vi "DependencyViewer_Configuration.vi"(8 "error in":errorcluster, 11 "ProjectPath":path) -> (0 "error out":errorcluster)   [LabVIEW 2020]
uses:
  DependencyChecker/FilterOptions.ctl
  DependencyChecker/Settings.ctl
  DependencyChecker/DependencyConfiguration.ctl
  <vilib>/Utility/sysdir.llb/System Directory Type.ctl
  DP-Common/DP-Common.lvlib
  DependencyViewer/DependencyViewer.lvlib
panel:
  in  "Max reports to save":u8 min=1
  in  "Close":bool
  in  "SaveChanges":bool
  in  "IgnoreLibrariesInCircularDependencies":bool
  in  "OnlyKeepCircularDepedencies":bool
  in  "Filter Options":T1={"Ignore user.lib"=FALSE, "Ignore vi.lib"=FALSE, "Ignore instr.lib"=FALSE, "FolderToIgnore"=[], "Ignore libraries"=FALSE, "Ignore lvcasses"=FALSE, "Ignore xnodes"=TRUE, "Ignore xcontrols"=TRUE, "Ignore Channel Classes"=TRUE}
  in  "RemoveEvenSubLibraries":bool
  in  "RemoveItemsBelongingToLibraries":bool
  in  "OpenFolder":bool
  in  "EmbedChartScript":bool
  in  "Remove Configuration":bool
  in  "Dependency configuration name":string
  in  "Add Configuration":bool
  in  "_ShowContextHelp":bool
  in  "Help":bool
  in  "Revert":bool
  in  "Update":bool
  in  "Dependency configurations":i32(listbox) caption="Will show up in the right click menu"
  in  "UseProjectFolder":bool
  in  "Folder to save reports to":path caption="Folder to save reports to (Absolute)"
  # "Dependency Viewer Configuration"
  # "Filter option for configuration"
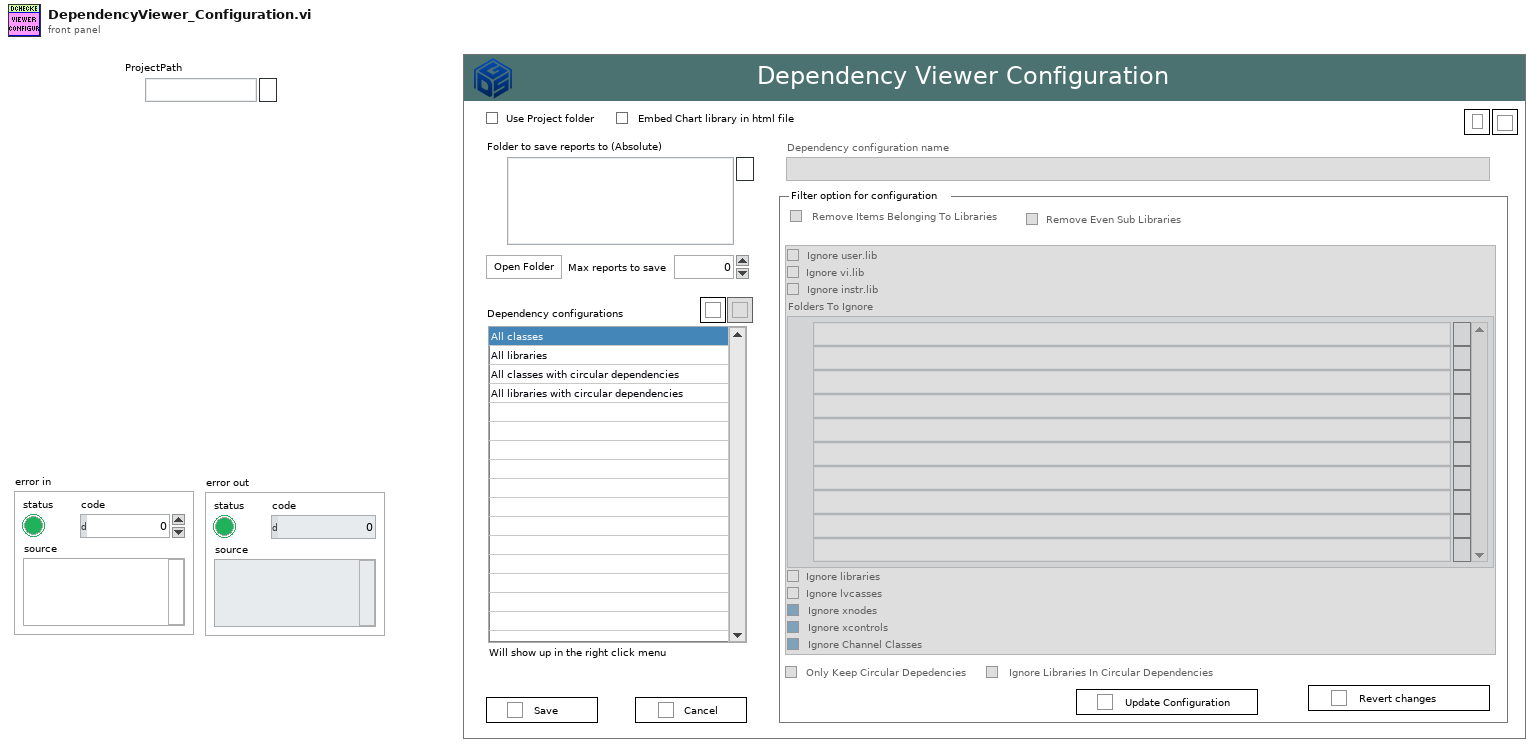
[diagram p1: front panel]
types:
  T1 = typedef "DependencyViewer.lvlib/FilterOptions.ctl" = cluster{"Ignore user.lib":bool, "Ignore vi.lib":bool, "Ignore instr.lib":bool, "FolderToIgnore":path[], "Ignore libraries":bool, "Ignore lvcasses":bool, "Ignore xnodes":bool, "Ignore xcontrols":bool, "Ignore Channel Classes":bool}
  T2 = typedef "System Directory Type.ctl" = i32
  T3 = typedef "DependencyViewer.lvlib/Settings.ctl" = cluster{"EmbedChartLibraryScript":bool, "Configurations":T4[], "UseProjectFolder":bool, "Folder to save reports to":path, "Max reports to save":u8}
  T4 = typedef "DependencyViewer.lvlib/DependencyConfiguration.ctl" = cluster{"Name":string, "RemoveItemsBelongingToLibraries":bool, "RemoveEvenSubLibraries":bool, "FilterOptions":T1, "OnlyKeepCircularDepedencies":bool, "IgnoreLibrariesInCircularDependencies":bool}
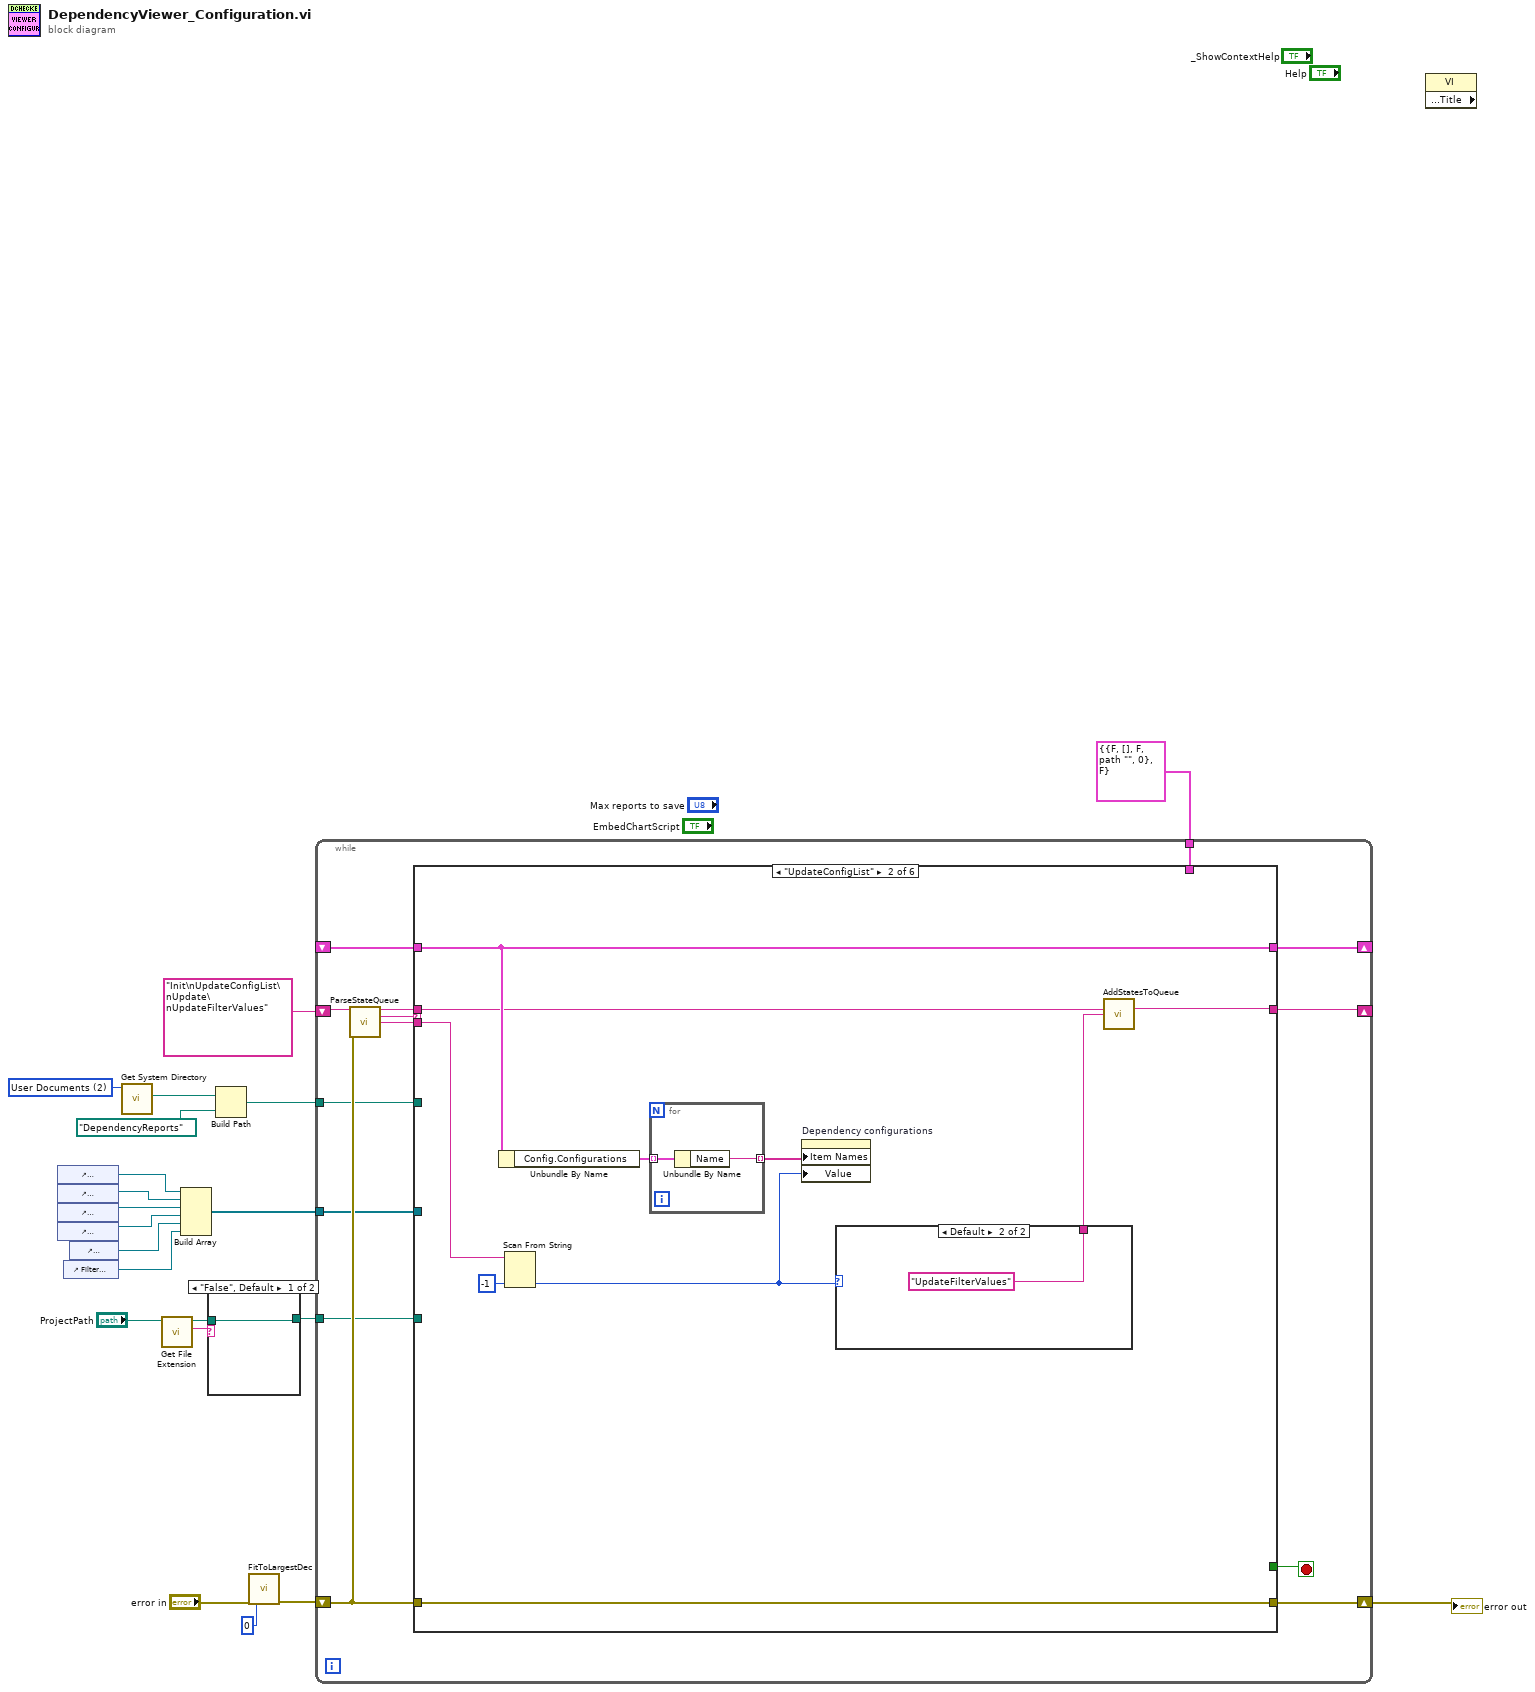
[diagram p0: block diagram]
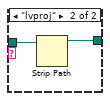
[diagram p2: hidden frame]
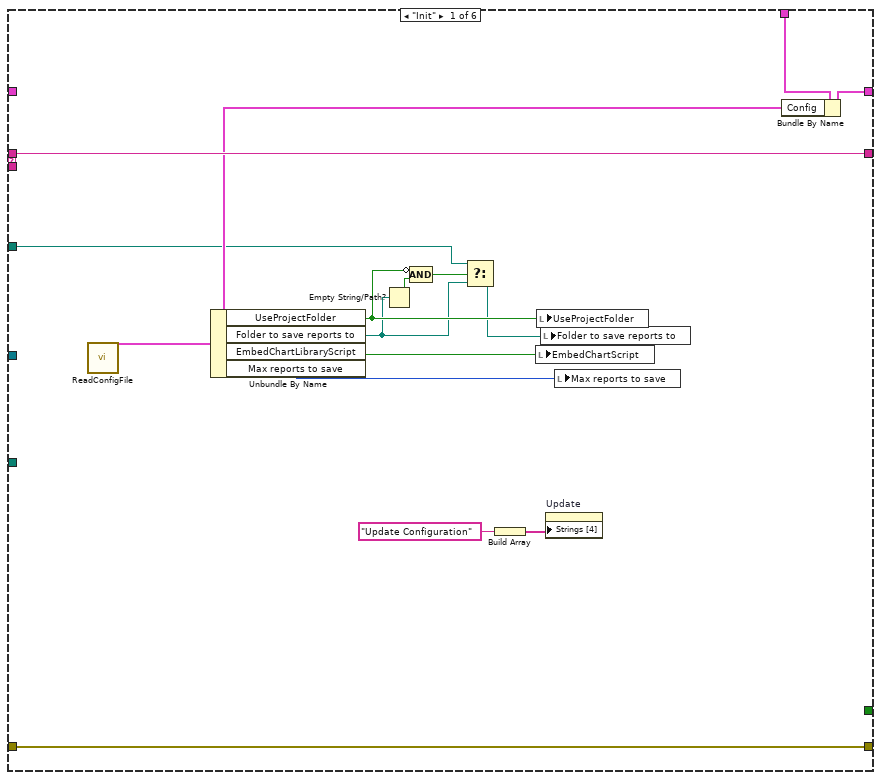
[diagram p3: hidden frame]
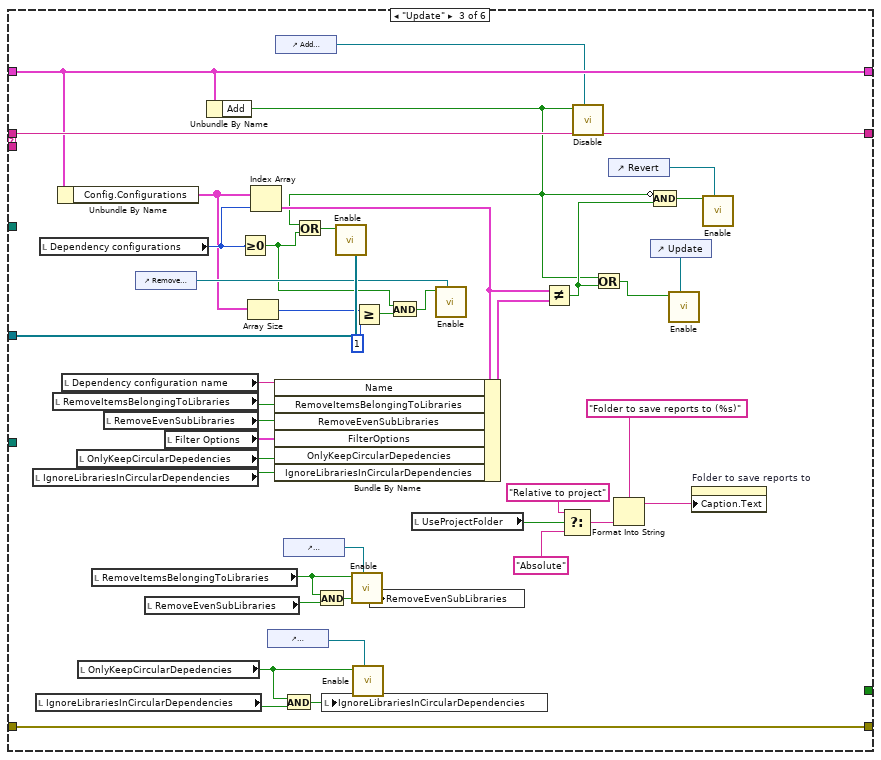
[diagram p5: hidden frame]
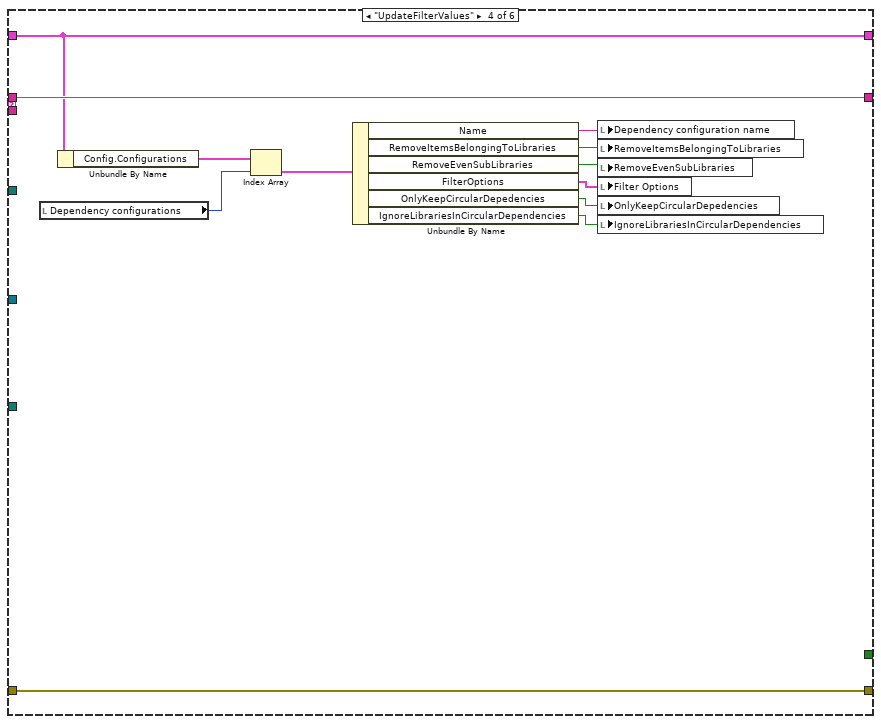
[diagram p6: hidden frame]
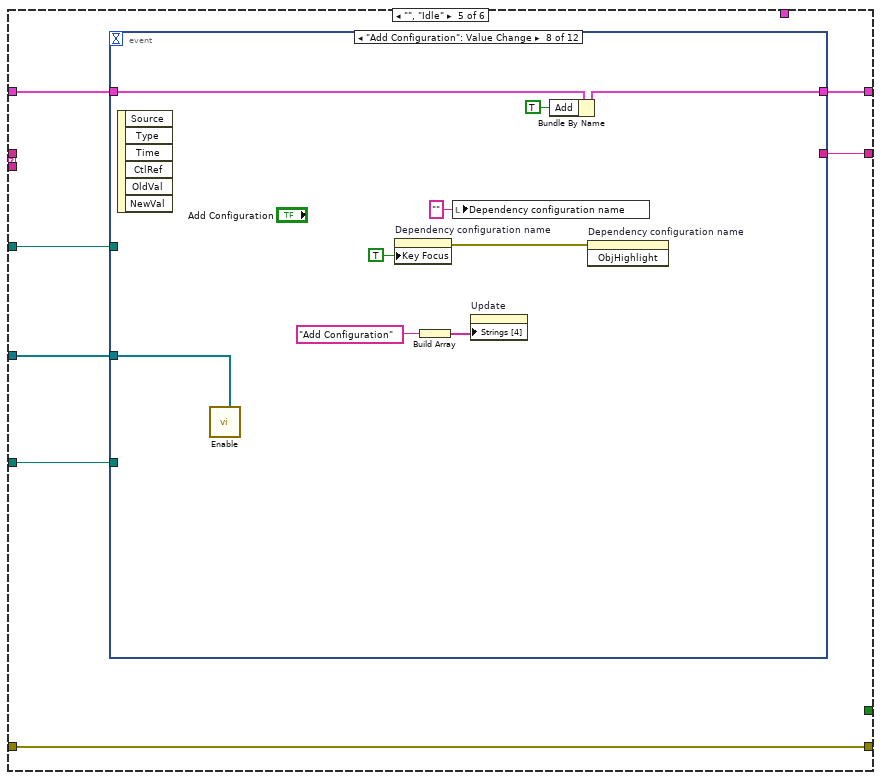
[diagram p7: hidden frame]
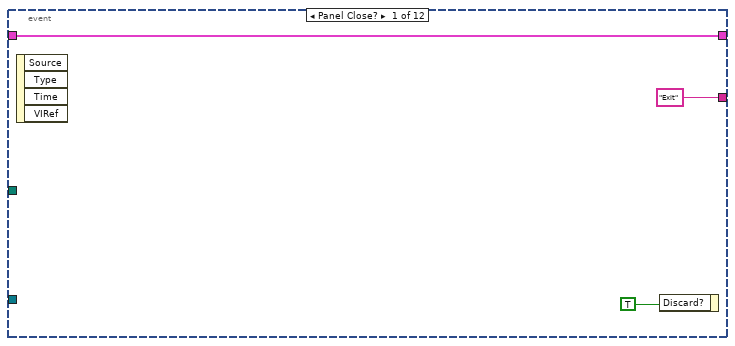
[diagram p8: hidden frame]
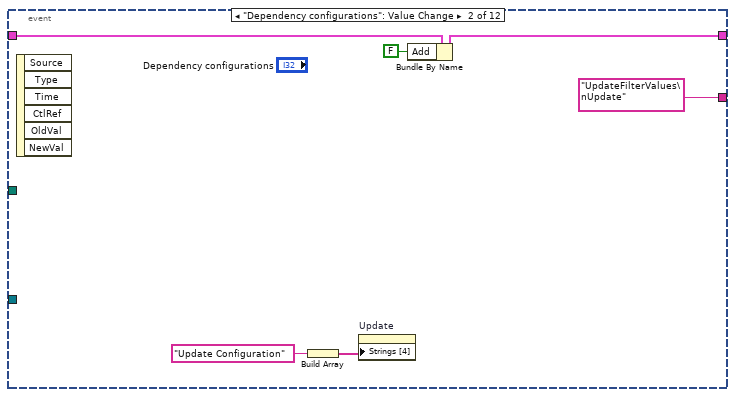
[diagram p9: hidden frame]
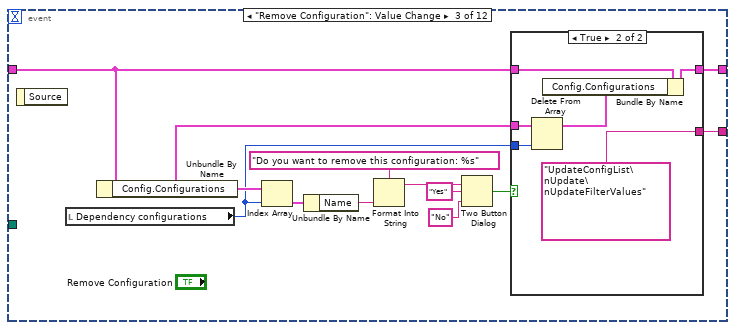
[diagram p10: hidden frame]
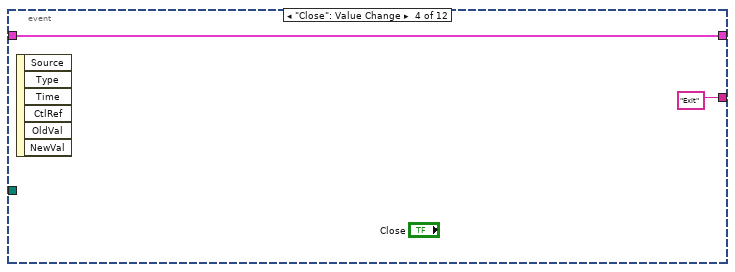
[diagram p12: hidden frame]
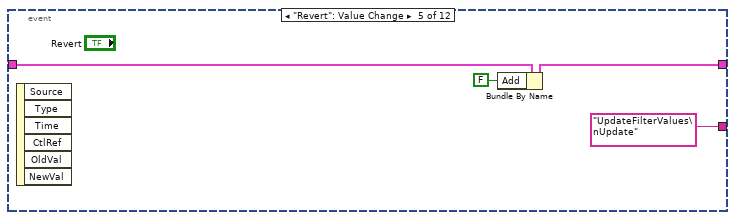
[diagram p13: hidden frame]
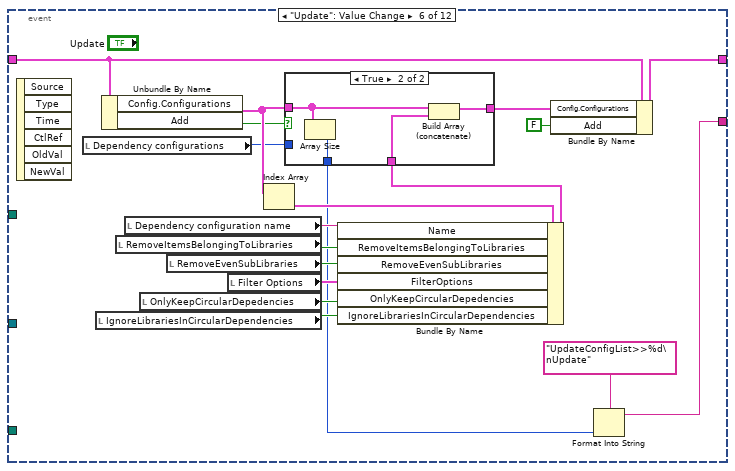
[diagram p14: hidden frame]
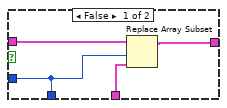
[diagram p15: hidden frame]
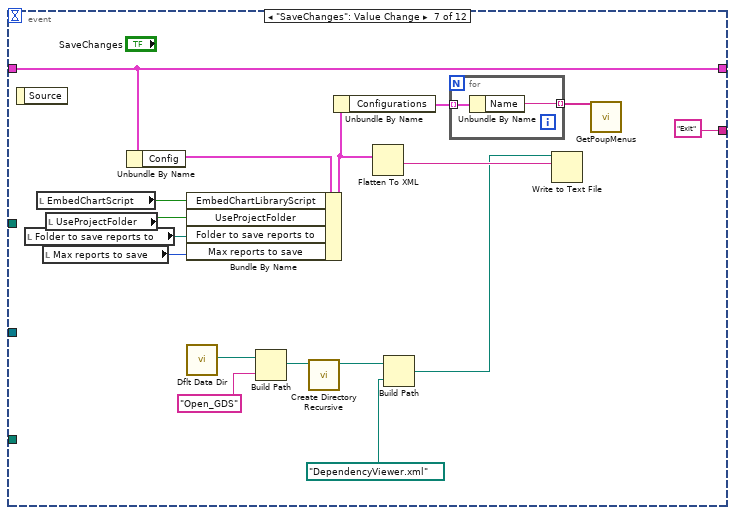
[diagram p16: hidden frame]
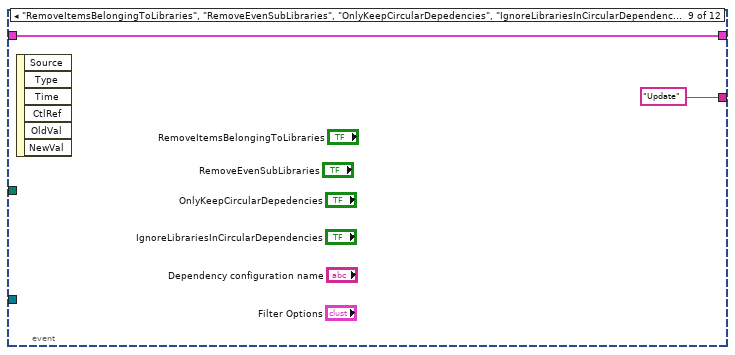
[diagram p17: hidden frame]
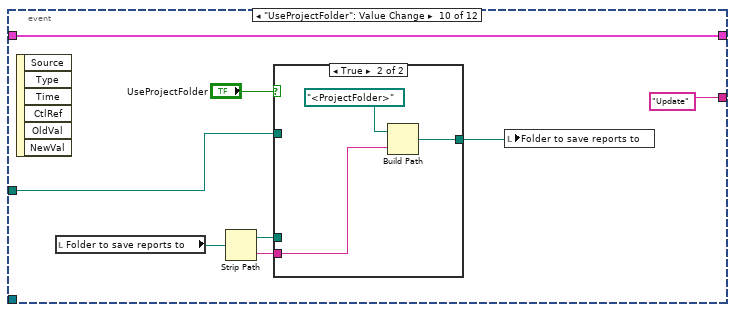
[diagram p18: hidden frame]
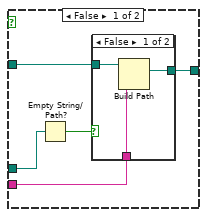
[diagram p19: hidden frame]
diagram:
  w8 = T2 2 items=["User Home"=0, "User Desktop"=1, "User Documents"=2, "User Application Data"=3, "User Preferences"=4, "User Temporary"=5, "Public Documents"=6, "Public Application Data"=7, "Public Preferences"=8, "Public Cache"=13, "System Core Libraries"=9, "System Installed Libraries"=10, "Application Files"=11, "Boot Volume Root"=12] ("system directory type")
  n1 = control-ref of="IgnoreLibrariesInCircularDependencies"() -> (w16:refnum<vi>)
  n2 = control-ref of="OnlyKeepCircularDepedencies"() -> (w15:refnum<vi>)
  n3 = control-ref of="RemoveEvenSubLibraries"() -> (w14:refnum<vi>)
  n4 = control-ref of="RemoveItemsBelongingToLibraries"() -> (w13:refnum<vi>)
  n5 = control-ref of="Filter Options"() -> (w11:refnum<vi>)
  n6 = control-ref of="Dependency configuration name"() -> (w12:refnum<vi>)
  n7 = call <vilib>:"Get System Directory.vi"("system directory type"=w8) -> ("system directory"=w7:path)  [unwired: 10 in]
  n8 = call <vilib>:"Get File Extension.vi"("file"="ProjectPath") -> ("lowercase file extension"=w3:string, "dup file"=w2:path)  [unwired: 6 in, 3 out]
  n9 = Build Array(w16, w15, w14, w13, w12, w11) -> (w10:refnum<vi>[])
  n10 = case shown="\"False\", Default" w3 {
    tunnel: w2 -> [w22 w24]
    tunnel: [w22 w23] -> w1
    frame "False", Default {
    }
    frame "lvproj" {
      n11 = Strip Path(path=w24) -> (stripped path=w23:path)  [unwired: 1 out]
    }
  }
  n12 = Build Path(base path=w7, name or relative path=path "DependencyReports") -> (appended path=w5:path)
  n13 = call "FitToLargestDec.vi"("error in (no error)"="error in", "border spacing (2 px)"=0) -> ("error out"=w17:errorcluster)  [unwired: 4 in, 1 out]
  n14 = while {
    shift-right: [w33] -> _
    shift-left: "Init\nUpdateConfigList\nUpdate\nUpdateFilterValues" -> [w38]
    shift-right: [w35] -> w19
    shift-left: w17 -> [w36]
    tunnel: cluster{"Config":T3, "Add":bool} {"Config"={"EmbedChartLibraryScript"=FALSE, "Configurations"=[], "UseProjectFolder"=FALSE, "Folder to save reports to"=path "", "Max reports to save"=0}, "Add"=FALSE} -> [w31]
    shift-right: [w30] -> _
    shift-left: _ -> [w29]
    tunnel: w10 -> [w27]
    tunnel: w5 -> [w26]
    tunnel: w1 -> [w25]
    stop <- w32 stop-if-true
    n15 = call "ParseStateQueue.vi"("State Queue"=w38, "Error In (no error)"=w36) -> ("Remaining States"=w34:string, "Current State"=w37:string, "Arguments"=w28:string)  [unwired: 9 in, 2 out]
    n16 = case shown="\"UpdateConfigList\"" w37 {
      tunnel: w36 -> [w53 w63 w99 w119 w127 w266]
      tunnel: [w53 w63 w99 w119 w127 w266] -> w35
      tunnel: [w52 w56 w100 w120 w124 w268] -> w33
      tunnel: w34 -> [w52 w57 w100 w120 _ w268]
      tunnel: [_ _ _ _ _ TRUE] -> w32
      tunnel: w31 -> [w51 _ _ _ _ _]
      tunnel: [w50 w61 w81 w118 w125 w265] -> w30
      tunnel: w29 -> [_ w61 w81 w118 w126 w265]
      tunnel: w28 -> [_ w59 _ _ _ _]
      tunnel: w27 -> [_ _ w97 _ w121 _]
      tunnel: w26 -> [w39 _ _ _ w123 _]
      tunnel: w25 -> [_ _ _ _ w122 _]
      frame "Init" {
        n17 = call "ReadConfigFile.vi"() -> ("Config"=w49:T3)  [unwired: 11 in]
        n18 = Unbundle By Name(w49) -> ("UseProjectFolder"=w44:bool, "Folder to save reports to"=w41:path, "EmbedChartLibraryScript"=w48:bool, "Max reports to save"=w45:u8)
        n19 = Empty String/Path?(string/path=w41) -> (empty?=w43:bool)
        n20 = Compound Arithmetic op=AND(invert w44, w43) -> (w42:bool)
        n21 = Select(t=w39, s=w42, f=w41) -> (s? t:f=w40:path)
        n22 = Build Array("Update Configuration") -> (w47:string[])
        n23 = local write "EmbedChartScript"(w48) -> ()
        n24 = local write "UseProjectFolder"(w44) -> ()
        n25 = local write "Folder to save reports to"(w40) -> ()
        n26 = property on="Update" class="Bool"("Strings [4]"=w47) -> ()  [unwired: 2 in, 2 out]
        n27 = local write "Max reports to save"(w45) -> ()
        n28 = Bundle By Name(cluster=w51, "Config"=w49) -> (w50:cluster{"Config":T3, "Add":bool})
      }
      frame "UpdateConfigList" {
        n29 = Unbundle By Name(w61) -> ("Config.Configurations"=w62:T4[])
        n30 = Scan From String(input string=w59, default 1=-1 ("default value 1")) -> (output 1=w55:i32)  [unwired: 3 in, 3 out]
        n31 = for {
          tunnel: w62 -> [w66] mode=indexing
          tunnel: [w65] -> w60 mode=indexing
          n32 = Unbundle By Name(w66) -> ("Name"=w65:string)
        }
        n33 = property on="Dependency configurations" class="LstBox (strict)"("Item Names"=w60, "Value"=w55) -> ()  [unwired: 2 in, 2 out]
        n34 = case shown="Default" w55 {
          tunnel: [_ "UpdateFilterValues"] -> w54
          frame -1 {
          }
          frame Default {
          }
        }
        n35 = call "AddStatesToQueue.vi"("State(s) in (\"\")"=w57, "State(s) at Back (\"\")"=w54) -> ("States Out"=w56:string)  [unwired: 13 in]
      }
      frame "Update" {
        n36 = local read "IgnoreLibrariesInCircularDependencies"() -> (w90:bool)
        n37 = local read "IgnoreLibrariesInCircularDependencies"() -> (w102:bool)
        n38 = local read "Dependency configurations"() -> (w98:i32)
        n39 = local read "RemoveItemsBelongingToLibraries"() -> (w94:bool)
        n40 = Unbundle By Name(w81) -> ("Config.Configurations"=w87:T4[])
        n41 = local read "Dependency configuration name"() -> (w95:string)
        n42 = local read "OnlyKeepCircularDepedencies"() -> (w91:bool)
        n43 = local read "OnlyKeepCircularDepedencies"() -> (w103:bool)
        n44 = local read "RemoveItemsBelongingToLibraries"() -> (w106:bool)
        n45 = local read "RemoveEvenSubLibraries"() -> (w93:bool)
        n46 = control-ref of="Remove Configuration"() -> (w96:refnum<vi>)
        n47 = local read "RemoveEvenSubLibraries"() -> (w107:bool)
        n48 = local read "Filter Options"() -> (w92:T1)
        n49 = Unbundle By Name(w81) -> ("Add"=w68:bool)
        n50 = Greater Or Equal To 0?(x=w98) -> (x >= 0?=w72:bool)
        n51 = Array Size(array=w87) -> (size(s)=w86:i32)
        n52 = Index Array(array=w87, index=w98) -> (element=w88:T4)
        n53 = control-ref of="IgnoreLibrariesInCircularDependencies"() -> (w104:refnum<vi>)
        n54 = Bundle By Name(cluster=w88, "Name"=w95, "RemoveItemsBelongingToLibraries"=w94, "RemoveEvenSubLibraries"=w93, "FilterOptions"=w92, "OnlyKeepCircularDepedencies"=w91, "IgnoreLibrariesInCircularDependencies"=w90) -> (w89:T4)
        n55 = control-ref of="Add Configuration"() -> (w67:refnum<vi>)
        n56 = control-ref of="RemoveEvenSubLibraries"() -> (w108:refnum<vi>)
        n57 = And(x=w103, y=w102) -> (x .and. y?=w101:bool)
        n58 = Or(x=w68, y=w72) -> (x .or. y?=w71:bool)
        n59 = And(x=w106, y=w107) -> (x .and. y?=w105:bool)
        n60 = local write "IgnoreLibrariesInCircularDependencies"(w101) -> ()
        n61 = call "Enable.vi"("ManyControls"=w97, "Enable(True)"=w71) -> ()  [unwired: 9 in, 1 out]
        n62 = call "Enable.vi"("ControlRefnum(IgnoreIfNotWired)"=w108, "Enable(True)"=w106) -> ()  [unwired: 9 in, 1 out]
        n63 = call "Enable.vi"("ControlRefnum(IgnoreIfNotWired)"=w104, "Enable(True)"=w103) -> ()  [unwired: 9 in, 1 out]
        n64 = Greater Or Equal?(x=w86, y=1) -> (x >= y?=w84:bool)
        n65 = local write "RemoveEvenSubLibraries"(w105) -> ()
        n66 = And(x=w72, y=w84) -> (x .and. y?=w83:bool)
        n67 = local read "UseProjectFolder"() -> (w77:bool)
        n68 = call "Enable.vi"("ControlRefnum(IgnoreIfNotWired)"=w96, "Enable(True)"=w83) -> ()  [unwired: 9 in, 1 out]
        n69 = Not Equal?(x=w88, y=w89) -> (x != y?=w70:bool)
        n70 = Select(t="Relative to project", s=w77, f="Absolute") -> (s? t:f=w76:string)
        n71 = call "Disable.vi"("ControlRefnum(IgnoreIfNotWired)"=w67, "Disasble(True)"=w68) -> ()  [unwired: 9 in, 1 out]
        n72 = Or(x=w68, y=w70) -> (x .or. y?=w69:bool)
        n73 = control-ref of="Revert"() -> (w79:refnum<vi>)
        n74 = Format Into String(format string="Folder to save reports to (%s)", w76) -> (resulting string=w75:string)  [unwired: 2 in, 1 out]
        n75 = control-ref of="Update"() -> (w82:refnum<vi>)
        n76 = Compound Arithmetic op=AND(invert w68, w70) -> (w80:bool)
        n77 = call "Enable.vi"("ControlRefnum(IgnoreIfNotWired)"=w82, "Enable(True)"=w69) -> ()  [unwired: 9 in, 1 out]
        n78 = property on="Folder to save reports to" class="Path"("Caption.Text"=w75) -> ()  [unwired: 2 in, 2 out]
        n79 = call "Enable.vi"("ControlRefnum(IgnoreIfNotWired)"=w79, "Enable(True)"=w80) -> ()  [unwired: 9 in, 1 out]
      }
      frame "UpdateFilterValues" {
        n80 = local read "Dependency configurations"() -> (w116:i32)
        n81 = Unbundle By Name(w118) -> ("Config.Configurations"=w117:T4[])
        n82 = Index Array(array=w117, index=w116) -> (element=w115:T4)
        n83 = Unbundle By Name(w115) -> ("Name"=w114:string, "RemoveItemsBelongingToLibraries"=w113:bool, "RemoveEvenSubLibraries"=w112:bool, "FilterOptions"=w111:T1, "OnlyKeepCircularDepedencies"=w110:bool, "IgnoreLibrariesInCircularDependencies"=w109:bool)
        n84 = local write "Dependency configuration name"(w114) -> ()
        n85 = local write "RemoveItemsBelongingToLibraries"(w113) -> ()
        n86 = local write "RemoveEvenSubLibraries"(w112) -> ()
        n87 = local write "Filter Options"(w111) -> ()
        n88 = local write "OnlyKeepCircularDepedencies"(w110) -> ()
        n89 = local write "IgnoreLibrariesInCircularDependencies"(w109) -> ()
      }
      frame "", "Idle" {
        n90 = event shown="[7] \"Add Configuration\": Value Change" {
          selector: _ -> [_ _ _ _ _ _ _ _ _ _ _ _]
          dyn-events: _ -> [_ _ _ _ _ _ _ _ _ _ _ _]
          timeout: _ -> [_ _ _ _ _ _ _ _ _ _ _ _]
          tunnel: w126 -> [w130 w135 w139 w157 w161 w173 w203 w215 w217 w225 w245 w261]
          tunnel: [w130 w132 w141 w157 w159 w172 w203 w211 w217 w225 w245 w261] -> w125
          tunnel: ["Exit" "UpdateFilterValues\nUpdate" w137 "Exit" "UpdateFilterValues\nUpdate" w163 "Exit" _ "Update" "Update" _ _] -> w124
          tunnel: w123 -> [_ _ _ _ _ _ _ _ _ w219 _ _]
          tunnel: w122 -> [_ _ _ _ _ _ _ _ _ _ w240 _]
          tunnel: w121 -> [_ _ _ _ _ _ _ w212 _ _ _ _]
          event Panel Close? {
            n91 = event-data() -> ()  [unwired: 1 in, 4 out]
            n92 = event-data("Discard?"=TRUE) -> ()  [unwired: 1 in, 1 out]
          }
          event "Dependency configurations": Value Change {
            n93 = event-data() -> ()  [unwired: 1 in, 6 out]
            n94 = Build Array("Update Configuration") -> (w134:string[])
            n95 = property on="Update" class="Bool"("Strings [4]"=w134) -> ()  [unwired: 2 in, 2 out]
            n96 = Bundle By Name(cluster=w135, "Add"=FALSE) -> (w132:cluster{"Config":T3, "Add":bool})
          }
          event "Remove Configuration": Value Change {
            n97 = event-data() -> ()  [unwired: 1 in, 1 out]
            n98 = local read "Dependency configurations"() -> (w138:i32)
            n99 = Unbundle By Name(w139) -> ("Config.Configurations"=w140:T4[])
            n100 = Index Array(array=w140, index=w138) -> (element=w148:T4)
            n101 = Unbundle By Name(w148) -> ("Name"=w146:string)
            n102 = Format Into String(format string="Do you want to remove this configuration: %s", w146) -> (resulting string=w145:string)  [unwired: 2 in, 1 out]
            n103 = Two Button Dialog(message=w145, 1:"No" ("T button name (\"OK\")"), 2:"Yes" ("T button name (\"OK\")")) -> (T button?=w142:bool)
            n104 = case shown="True" w142 {
              tunnel: [w149 w152] -> w141
              tunnel: w140 -> [_ w155]
              tunnel: w139 -> [w149 w154]
              tunnel: w138 -> [_ w151]
              tunnel: [_ "UpdateConfigList\nUpdate\nUpdateFilterValues"] -> w137
              frame False {
              }
              frame True {
                n105 = Delete From Array(array=w155, index=w151) -> (array with subset deleted=w153:T4[])  [unwired: 1 in, 1 out]
                n106 = Bundle By Name(cluster=w154, "Config.Configurations"=w153) -> (w152:cluster{"Config":T3, "Add":bool})
              }
            }
          }
          event "Close": Value Change {
            n107 = event-data() -> ()  [unwired: 1 in, 6 out]
          }
          event "Revert": Value Change {
            n108 = event-data() -> ()  [unwired: 1 in, 6 out]
            n109 = Bundle By Name(cluster=w161, "Add"=FALSE) -> (w159:cluster{"Config":T3, "Add":bool})
          }
          event "Update": Value Change {
            n110 = event-data() -> ()  [unwired: 1 in, 6 out]
            n111 = local read "Dependency configurations"() -> (w166:i32)
            n112 = local read "IgnoreLibrariesInCircularDependencies"() -> (w174:bool)
            n113 = Unbundle By Name(w173) -> ("Config.Configurations"=w169:T4[], "Add"=w167:bool)
            n114 = local read "RemoveItemsBelongingToLibraries"() -> (w178:bool)
            n115 = local read "Dependency configuration name"() -> (w179:string)
            n116 = local read "OnlyKeepCircularDepedencies"() -> (w175:bool)
            n117 = local read "RemoveEvenSubLibraries"() -> (w177:bool)
            n118 = local read "Filter Options"() -> (w176:T1)
            n119 = Index Array(array=w169) -> (element=w168:T4)  [unwired: 1 in]
            n120 = Bundle By Name(cluster=w168, "Name"=w179, "RemoveItemsBelongingToLibraries"=w178, "RemoveEvenSubLibraries"=w177, "FilterOptions"=w176, "OnlyKeepCircularDepedencies"=w175, "IgnoreLibrariesInCircularDependencies"=w174) -> (w171:T4)
            n121 = case shown="True" w167 {
              tunnel: w171 -> [w181 w187]
              tunnel: [w182 w186] -> w170
              tunnel: w169 -> [w183 w185]
              tunnel: w166 -> [w180 _]
              tunnel: [w180 w184] -> w162
              frame False {
                n122 = Replace Array Subset(array=w183, new element=w181, index=w180) -> (w182:T4[])
              }
              frame True {
                n123 = Array Size(array=w185) -> (size(s)=w184:i32)
                n124 = Build Array (concatenate)(w185, w187) -> (w186:T4[])
              }
            }
            n125 = Bundle By Name(cluster=w173, "Config.Configurations"=w170, "Add"=FALSE) -> (w172:cluster{"Config":T3, "Add":bool})
            n126 = Format Into String(format string="UpdateConfigList>>%d\nUpdate", w162) -> (resulting string=w163:string)  [unwired: 2 in, 1 out]
          }
          event "SaveChanges": Value Change {
            n127 = event-data() -> ()  [unwired: 1 in, 1 out]
            n128 = local read "Folder to save reports to"() -> (w193:path)
            n129 = local read "EmbedChartScript"() -> (w195:bool)
            n130 = local read "Max reports to save"() -> (w192:u8)
            n131 = local read "UseProjectFolder"() -> (w194:bool)
            n132 = Unbundle By Name(w203) -> ("Config"=w199:T3)
            n133 = Bundle By Name(cluster=w199, "EmbedChartLibraryScript"=w195, "UseProjectFolder"=w194, "Folder to save reports to"=w193, "Max reports to save"=w192) -> (w198:T3)
            n134 = call <vilib>:"Dflt Data Dir.vi"() -> ("App:Default Data Directory"=w190:path)
            n135 = Build Path(base path=w190, name or relative path="Open_GDS") -> (appended path=w189:path)
            n136 = call <vilib>:"Create Directory Recursive.vi"("directory"=w189) -> ("directory copy"=w188:path)  [unwired: 4 in, 2 out]
            n137 = Unbundle By Name(w198) -> ("Configurations"=w197:T4[])
            n138 = Flatten To XML(6:w198) -> (2:w201:string)
            n139 = Build Path(base path=w188, name or relative path=path "DependencyViewer.xml") -> (appended path=w200:path)
            n140 = for {
              tunnel: [w206] -> w196 mode=indexing
              tunnel: w197 -> [w205] mode=indexing
              n141 = Unbundle By Name(w205) -> ("Name"=w206:string)
            }
            n142 = Write to Text File(file (use dialog)=w200, text=w201) -> ()  [unwired: 2 in, 3 out]
            n143 = call "GetPoupMenus.vi"("Configurations"=w196) -> ()  [unwired: 10 in, 1 out]
          }
          event "Add Configuration": Value Change {
            n144 = event-data() -> ()  [unwired: 1 in, 6 out]
            n145 = call "Enable.vi"("ManyControls"=w212) -> ()  [unwired: 10 in, 1 out]
            n146 = property on="Dependency configuration name" class="Str"("Key Focus"=TRUE ("Add")) -> (error out=w207:errorcluster)  [unwired: 2 in, 1 out]
            n147 = Build Array("Add Configuration") -> (w214:string[])
            n148 = local write "Dependency configuration name"("" ("Dependency configuration name")) -> ()
            n149 = property on="Update" class="Bool"("Strings [4]"=w214) -> ()  [unwired: 2 in, 2 out]
            n150 = Bundle By Name(cluster=w215, "Add"=TRUE) -> (w211:cluster{"Config":T3, "Add":bool})
            n151 = invoke on="Dependency configuration name" class="Str" method="ObjHighlight"(error in=w207) -> ()  [unwired: 2 in, 3 out]
          }
          event "RemoveItemsBelongingToLibraries", "RemoveEvenSubLibraries", "OnlyKeepCircularDepedencies", "IgnoreLibrariesInCircularDependencies", "Dependency configuration name": Value Change {
            n152 = event-data() -> ()  [unwired: 1 in, 6 out]
          }
          event "UseProjectFolder": Value Change {
            n153 = event-data() -> ()  [unwired: 1 in, 6 out]
            n154 = local read "Folder to save reports to"() -> (w222:path)
            n155 = Strip Path(path=w222) -> (stripped path=w218:path, name=w221:string)
            n156 = case shown="True" "UseProjectFolder" {
              tunnel: w221 -> [w226 w236]
              tunnel: [w227 w235] -> w220
              tunnel: w219 -> [w230 _]
              tunnel: w218 -> [w229 _]
              frame False {
                n157 = Empty String/Path?(string/path=w229) -> (empty?=w228:bool)
                n158 = case shown="False" w228 {
                  tunnel: w230 -> [w233 w234]
                  tunnel: [w231 w234] -> w227
                  tunnel: w226 -> [w232 _]
                  frame False {
                    n159 = Build Path(base path=w233, name or relative path=w232) -> (appended path=w231:path)
                  }
                  frame True {
                  }
                }
              }
              frame True {
                n160 = Build Path(base path=path "<ProjectFolder>", name or relative path=w236) -> (appended path=w235:path)
              }
            }
            n161 = local write "Folder to save reports to"(w220) -> ()
          }
          event "OpenFolder": Value Change {
            n162 = event-data() -> ()  [unwired: 1 in, 6 out]
            n163 = local read "Folder to save reports to"() -> (w242:path)
            n164 = local read "UseProjectFolder"() -> (w243:bool)
            n165 = case shown="True" w243 {
              tunnel: w242 -> [w246 w250]
              tunnel: [w246 w247] -> w239
              tunnel: w240 -> [_ w249]
              frame False {
              }
              frame True {
                n166 = Strip Path(path=w250) -> (name=w248:string)  [unwired: 1 out]
                n167 = Build Path(base path=w249, name or relative path=w248) -> (appended path=w247:path)
              }
            }
            n168 = call <vilib>:"Create Directory Recursive.vi"("directory"=w239) -> ("directory copy"=w238:path)  [unwired: 4 in, 2 out]
            n169 = Format Into String(format string="explorer \"%s\"", w238) -> (resulting string=w241:string)  [unwired: 2 in, 1 out]
            n170 = call <vilib>:"System Exec.vi"("command line"=w241) -> ()  [unwired: 7 in, 4 out]
          }
          event "Folder to save reports to": Value Change {
            n171 = event-data() -> ()  [unwired: 1 in, 6 out]
            n172 = Path Type(1:"Folder to save reports to") -> (0:w258:i16)
            n173 = Strip Path(path="Folder to save reports to") -> (name=w260:string)  [unwired: 1 out]
            n174 = Equal?(x=w258, y=i16 1) -> (x = y?=w254:bool)
            n175 = Match Pattern(string=w260, regular expression="<") -> (offset past match=w256:i32)  [unwired: 1 in, 3 out]
            n176 = Greater Or Equal To 0?(x=w256) -> (x >= 0?=w253:bool)
            n177 = Compound Arithmetic op=AND(w254, invert w253) -> (w252:bool)
            n178 = Or(x=w254, y=w253) -> (x .or. y?=w255:bool)
            n179 = case shown="True" w252 {
              tunnel: "Folder to save reports to" -> [_ w263]
              frame False {
              }
              frame True {
                n180 = Build Path(base path=path "<ProjectFolder>", name or relative path=w263) -> (appended path=w262:path)
                n181 = local write "Folder to save reports to"(w262) -> ()
              }
            }
            n182 = local write "UseProjectFolder"(w255) -> ()
          }
        }
      }
      frame "Error", "Exit", Default {
      }
    }
  }
  "error out" <- w19
  n183 = property class="VI" props=["Front Panel.Title"]() -> ()  [unwired: 2 in, 3 out]
